vi "sv_Convert Complex Spectrum.vi"(0 "complex spectrum":T7={"complex spectrum response"={"f0"=0.0, "df"=1.0, "complex spectrum"=[]}, "spectrum info"={"channel name"="", "description"="", "x-axis units"=0, "spectral info"={"spectrum type"=enum."Power [Magnitude^2]", "linear/dB"=enum."linear", "window"=0, "window size"=0, "FFT size"=0}, "engineering units"=0, "custom label"="", "dB reference [EU]"=0.0, "peak units"=enum."rms", "weighting filter"=0, "spectral density?"=FALSE, "unit label"="", "spectrum skewed?"=FALSE, "complimentary spectrum units"=enum."none"}} {"spectrum info"."x-axis units" items=["time"=0, "frequency"=1, "quefrency"=2, "revolutions"=3, "order"=4, "rpm"=11, "rad/s"=21, "index"=65535]; "spectrum info"."weighting filter" items=["Linear", "A-weighting", "B-weighting", "C-weighting", "ITU-R 468-4", "Dolby", "CCITT", "C-message"]; "spectrum info"."dB reference [EU]" format="%.2f"; "spectrum info"."engineering units" items=["custom..."=0, "V"=1, "A"=21, "Pa"=2, "N"=20, "g"=3, "m/s^2"=4, "m/s"=5, "m"=6, "mm/s"=12, "mm"=13, "microns/s"=14, "microns"=15, "in/s^2"=7, "in/s"=8, "in"=9, "mils/s"=10, "mils"=11, "rad/s^2"=16, "rad/s"=17, "rad"=18, "strain"=19]; "spectrum info"."spectral info"."window" items=["None "=0, "Hanning"=1, "Hamming"=2, "Blackman-Harris"=3, "Exact Blackman"=4, "Blackman"=5, "Flat Top"=6, "4 Term B-Harris "=7, "7 Term B-Harris"=8, "Low Sidelobe"=9, "Force - Exponential"=10, "Gaussian"=62]; "complex spectrum response"."complex spectrum" format="%.2f"; "complex spectrum response"."df" format="%.2f"; "complex spectrum response"."f0" format="%.2f"}, 3 "view for \"Mag-Phase\" type":T1={"dB On (F)"=TRUE, "unwrap phase (F)"=FALSE, "convert to degree (T)"=TRUE}, 5 "error in":errorcluster, 6 "output spectrum type":enum16{"Mag-Phase", "Real-Imaginary"}(ring)) -> (14 "magnitude or real":cluster{"f0":dbl, "df":dbl, "magnitude":dbl[]} {"magnitude" format="%.2p"; "df" format="%.2p"; "f0" format="%.2p"}, 15 "unit label [mag or real]":string, 16 "phase or imaginary":cluster{"f0":dbl, "df":dbl, "phase":dbl[]} {"phase" format="%.2p"; "df" format="%.2p"; "f0" format="%.2p"}, 17 "unit label [phase or imag]":string, 18 "spectrum info":T2={"channel name"="", "description"="", "x-axis units"=0, "spectral info"={"spectrum type"=enum."Power [Magnitude^2]", "linear/dB"=enum."linear", "window"=0, "window size"=0, "FFT size"=0}, "engineering units"=0, "custom label"="", "dB reference [EU]"=0.0, "peak units"=enum."rms", "weighting filter"=0, "spectral density?"=FALSE, "unit label"="", "spectrum skewed?"=FALSE, "complimentary spectrum units"=enum."none"} {"x-axis units" items=["time"=0, "frequency"=1, "quefrency"=2, "revolutions"=3, "order"=4, "rpm"=11, "rad/s"=21, "index"=65535]; "weighting filter" items=["Linear", "A-weighting", "B-weighting", "C-weighting", "ITU-R 468-4", "Dolby", "CCITT", "C-message"]; "dB reference [EU]" format="%.2f"; "engineering units" items=["custom..."=0, "V"=1, "A"=21, "Pa"=2, "N"=20, "g"=3, "m/s^2"=4, "m/s"=5, "m"=6, "mm/s"=12, "mm"=13, "microns/s"=14, "microns"=15, "in/s^2"=7, "in/s"=8, "in"=9, "mils/s"=10, "mils"=11, "rad/s^2"=16, "rad/s"=17, "rad"=18, "strain"=19]; "spectral info"."window" items=["None "=0, "Hanning"=1, "Hamming"=2, "Blackman-Harris"=3, "Exact Blackman"=4, "Blackman"=5, "Flat Top"=6, "4 Term B-Harris "=7, "7 Term B-Harris"=8, "Low Sidelobe"=9, "Force - Exponential"=10, "Gaussian"=62]}, 19 "error out":errorcluster)   [LabVIEW 2017]
uses:
  <vilib>/addons/Sound and Vibration/compatibility/Controls/svl_Spectrum Info (enhanced).ctl
  <vilib>/addons/Sound and Vibration/compatibility/Controls/svl_Spectrum Type.ctl
  <vilib>/addons/Sound and Vibration/compatibility/Controls/svl_Engineering Units Text Ring.ctl
  <vilib>/addons/Sound and Vibration/compatibility/Controls/svl_Weighting Filter Text Ring.ctl
  <vilib>/addons/Sound and Vibration/compatibility/Controls/svl_Complimentary Spectrum Units.ctl
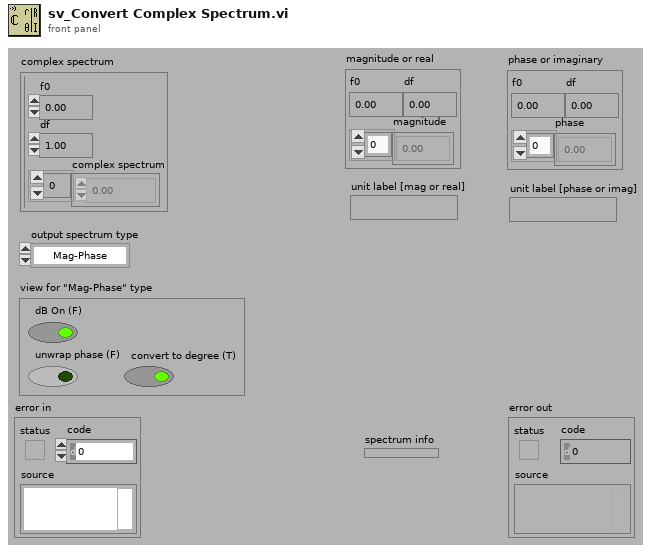
[diagram p1: front panel]
types:
  T1 = cluster{"dB On (F)":bool, "unwrap phase (F)":bool, "convert to degree (T)":bool}
  T2 = typedef "svl_Spectrum Info (enhanced).ctl" = cluster{"channel name":string, "description":string, "x-axis units":u16, "spectral info":cluster{"spectrum type":T3, "linear/dB":enum16{"linear", "dB"}, "window":u16, "window size":i32, "FFT size":i32}, "engineering units":T4, "custom label":string, "dB reference [EU]":dbl, "peak units":enum16{"rms", "peak", "peak-peak"}, "weighting filter":T5, "spectral density?":bool, "unit label":string, "spectrum skewed?":bool, "complimentary spectrum units":T6}
  T3 = typedef "svl_Spectrum Type.ctl" = enum16{"FFT Spectrum [complex]", "Amplitude [Magnitude]", "Power [Magnitude^2]", "Cross Spectrum [complex]", "Frequency Response [Complex]"}
  T4 = typedef "svl_Engineering Units Text Ring.ctl" = u16
  T5 = typedef "svl_Weighting Filter Text Ring.ctl" = u16
  T6 = typedef "svl_Complimentary Spectrum Units.ctl" = enum16{"none", "radians", "degrees", "cycles", "imaginary"}
  T7 = cluster{"complex spectrum response":cluster{"f0":dbl, "df":dbl, "complex spectrum":cdb[]}, "spectrum info":T2}
  T8 = enum16{"FFT Spectrum [complex]", "Amplitude [Magnitude]", "Power [Magnitude^2]", "Cross Spectrum [complex]", "Frequency Response [Complex]"}
  T9 = cluster{"f0":dbl, "df":dbl, "complex spectrum":cdb[]}
  T10 = typedef "svc_Spectrum Info.ctl" = cluster{"channel name":string, "description":string, "x-axis units":T11, "spectral info":cluster{"spectrum type":T12, "linear/dB":enum16{"linear", "dB"}, "window":u16, "window size":i32, "FFT size":i32}, "engineering units":T13, "custom label":string, "dB reference [EU]":dbl, "peak units":enum16{"rms", "peak", "peak-peak"}, "weighting filter":T14, "spectral density?":bool, "unit label":string, "spectrum skewed?":bool, "complimentary spectrum units":T15}
  T11 = typedef "svc_X-Axis Units.ctl" = u16
  T12 = typedef "svc_Spectrum Type.ctl" = enum16{"FFT Spectrum [complex]", "Amplitude [Magnitude]", "Power [Magnitude^2]", "Cross Spectrum [complex]", "Frequency Response [Complex]"}
  T13 = typedef "svc_Engineering Units Text Ring.ctl" = u16
  T14 = typedef "svc_Weighting Filter Text Ring.ctl" = u16
  T15 = typedef "svc_Complimentary Spectrum Units.ctl" = enum16{"none", "radians", "degrees", "cycles", "imaginary"}
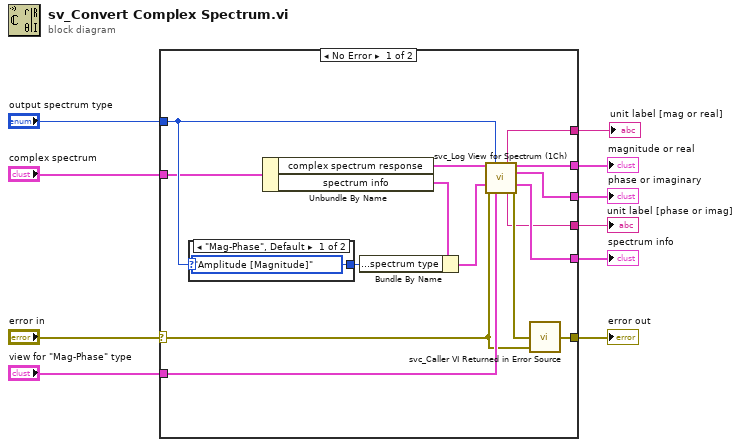
[diagram p0: block diagram]
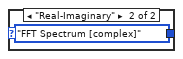
[diagram p2: hidden frame]
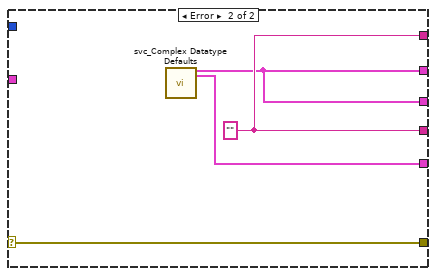
[diagram p3: hidden frame]
diagram:
  n1 = case shown="No Error" "error in" {
    selector: "error in" -> [w11 w31]
    tunnel: "output spectrum type" -> [w17 _]
    tunnel: [w24 w29] -> w9
    tunnel: [w20 w29] -> w8
    tunnel: "view for \"Mag-Phase\" type" -> [w23 _]
    tunnel: [w22 w31] -> w6
    tunnel: [w21 w28] -> w4
    tunnel: "complex spectrum" -> [w13 _]
    tunnel: [w19 w30] -> w2
    tunnel: [w18 w30] -> w1
    frame No Error {
      n2 = case shown="\"Mag-Phase\", Default" w17 {
        tunnel: [T8."Amplitude [Magnitude]" ("spectral info.spectrum type") T8."FFT Spectrum [complex]" ("spectral info.spectrum type")] -> w16
        frame "Mag-Phase", Default {
        }
        frame "Real-Imaginary" {
        }
      }
      n3 = Unbundle By Name(w13) -> ("complex spectrum response"=w12:T9, "spectrum info"=w14:T2)
      n4 = Bundle By Name(cluster=w14, "spectral info.spectrum type"=w16) -> (w15:T2)
      n5 = call <vilib>:"svc_Log View for Spectrum (1Ch).vi"("complex spectrum"=w12, "View"=w17, "spectrum info in"=w15, "error in (no error)"=w11, "view"=w23) -> ("unit label [mag or real]"=w19:string, "magnitude or real"=w24:cluster{"f0":dbl, "df":dbl, dbl[]}, "phase or imag"=w20:cluster{"f0":dbl, "df":dbl, dbl[]}, "spectrum info out"=w21:T10, "unit label [phase or imag]"=w18:string, "error out"=w25:errorcluster)  [unwired: 5 in]
      n6 = call <vilib>:"svc_Caller VI Returned in Error Source.vi"("warning input to caller"=w11, "error in (no error)"=w25) -> ("error out"=w22:errorcluster)  [unwired: 3 in]
    }
    frame Error {
      w30 = "" ("unit label [mag or real]")
      n7 = call <vilib>:"svc_Complex Datatype Defaults.vi"() -> ("empty spectrum"=w29:cluster{"f0":dbl, "df":dbl, "magnitude":dbl[]}, "dead spectrum info"=w28:T10)  [unwired: 11 in, 7 out]
    }
  }
  "error out" <- w6
  "magnitude or real" <- w9
  "phase or imaginary" <- w8
  "spectrum info" <- w4
  "unit label [phase or imag]" <- w1
  "unit label [mag or real]" <- w2
